vi "FileIndexToDiscIndex.vi"(10 "FileIndex":i32, 11 "FileData":u8[](array[numeric])) -> (3 "DiscIndees":u64)   [LabVIEW 2023, in "2024_9.lvclass"]
uses:
  2024_9.lvclass
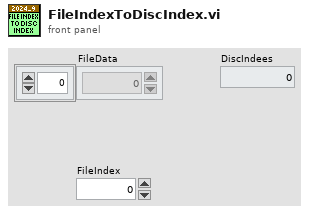
[diagram p1: front panel]
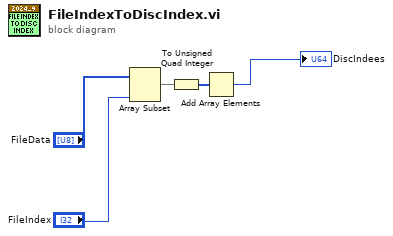
[diagram p0: block diagram]
diagram:
  n1 = Array Subset(array="FileData", length="FileIndex") -> (w3:u8[])  [unwired: 1 in]
  n2 = To Unsigned Quad Integer(1:w3) -> (0:w4:u64[])
  n3 = Add Array Elements(numeric array=w4) -> (sum=→"DiscIndees":u64)
